vi "GaGe4_GetSystem.vi"(8 "error in (no error)":errorcluster, 9 "Board index":i16 min=0 max=64 step=1, 10 "Board Name (Any)":string="any") -> (0 "error out":errorcluster, 3 "Handle Cluster out":T1)   [LabVIEW 2015]
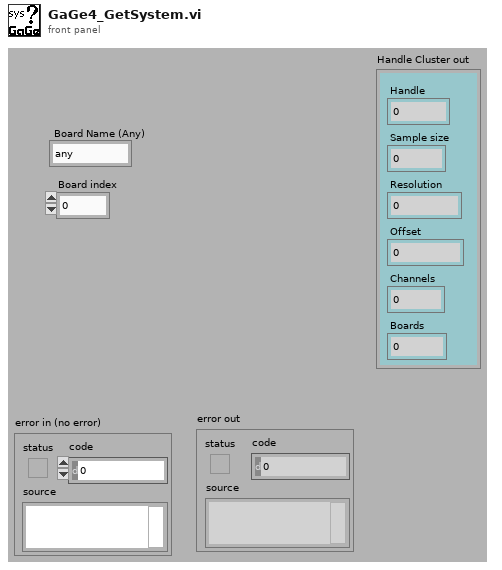
[diagram p1: front panel]
types:
  T1 = cluster{"Handle":u32, "Sample size":u32, "Resolution":i32, "Offset":i32, "Channels":u32, "Boards":u32}
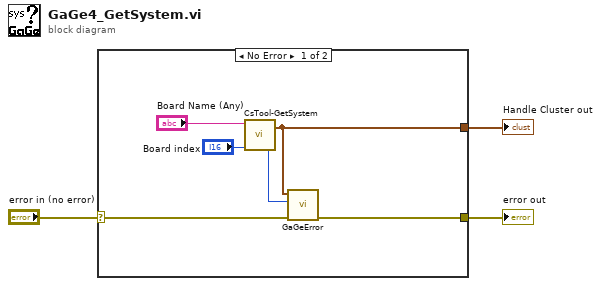
[diagram p0: block diagram]
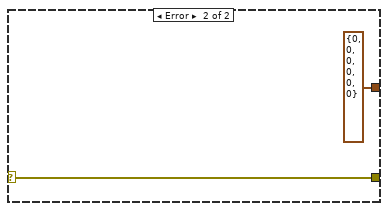
[diagram p2: hidden frame]
diagram:
  n1 = case shown="No Error" "error in (no error)" {
    selector: "error in (no error)" -> [w9 w11]
    tunnel: [w7 w11] -> w2
    tunnel: [w6 T1 {"Handle"=0, "Sample size"=0, "Resolution"=0, "Offset"=0, "Channels"=0, "Boards"=0} ("Handle Cluster")] -> w1
    frame No Error {
      n2 = call "CsTool-GetSystem.vi"("Index (0)"="Board index", "Board Name (Any)"="Board Name (Any)") -> ("Error Code"=w5:i32, "Handle Cluster"=w6:T1)  [unwired: 2 in]
      n3 = call "GaGeError.vi"("error in (no error)"=w9, "Error Code"=w5, "Handle Cluster"=w6) -> ("error out"=w7:errorcluster)  [unwired: 3 in, 5 out]
    }
    frame Error {
    }
  }
  "error out" <- w2
  "Handle Cluster out" <- w1
